vi "MFC_Setpoint.vi"(8 "error in (no error)":errorcluster, 10 "MFC set1":cluster{"String":string, "MFC set":dbl}[](array[cluster]) {"MFC set" format="%.3g"}, 11 "VISA Refnum in":refnum<visa-resource-name>="COM6") -> (0 "error out":errorcluster, 3 "VISA Refnum out":refnum<visa-resource-name>="COM6")   [LabVIEW 2014]
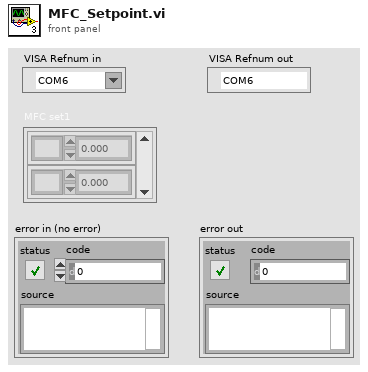
[diagram p1: front panel]
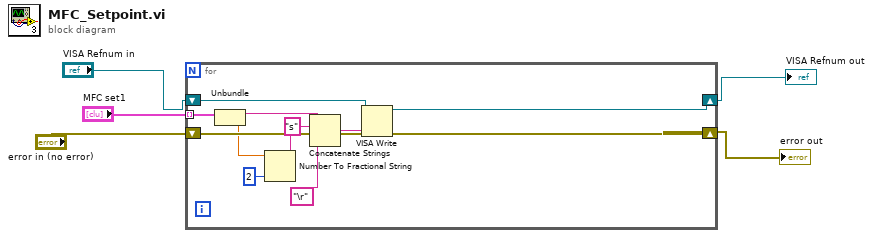
[diagram p0: block diagram]
diagram:
  n1 = for {
    shift-right: [w6] -> w4
    shift-left: "error in (no error)" -> [w17]
    shift-right: [w7] -> w5
    shift-left: "VISA Refnum in" -> [w16]
    tunnel: "MFC set1" -> [w13] mode=indexing
    n2 = Unbundle(w13) -> ("String"=w12:string, "MFC set"=w11:dbl)
    n3 = Number To Fractional String(number=w11, precision (6)=i16 2) -> (F-format string=w9:string)  [unwired: 2 in]
    n4 = Concatenate Strings(w12, "s" ("string"), w9, "\r" ("string")) -> (w15:string)
    n5 = VISA Write(VISA resource name=w16, write buffer=w15, error in (no error)=w17) -> (VISA resource name out=w7:refnum<visa-resource-name>, error out=w6:errorcluster)  [unwired: 1 out]
  }
  "VISA Refnum out" <- w5
  "error out" <- w4
